vi "Wrap Element To Display.vi"(10 "Camera":refnum<class "Camera.lvclass">, 11 "World Position":T1) -> (3 "Display Position":T1)   [LabVIEW 2018]
uses:
  Camera/Camera.lvclass
  LabSDL2/Source/Libraries/SDL2 Utility/Point (I32).ctl
  Camera/Camera.lvclass/Camera.ctl
  Math/Math.lvlib
  Globals.vi
  Element/Element.lvclass
  LabSDL2/Source/Libraries/SDL2 Utility/SDL2 Utility.lvlib
panel:
  in  "Point":T1
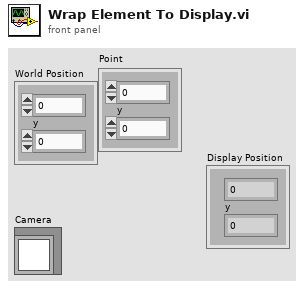
[diagram p1: front panel]
types:
  T1 = typedef "SDL2 Utility.lvlib/Point (I32).ctl" = cluster{"x":i32, "y":i32}
  T2 = typedef "Constants.ctl" = cluster{"Colours":cluster{"OK":u32, "Warning":u32, "Error":u32, "Red":u32, "Green":u32, "Blue":u32, "Yellow":u32}, "System":cluster{"Target Frames Second":dbl, "World Size":T1, "Window Size":T1, "Viewport Size":T1, "Sidebar Scaling":sgl, "Sidebar Width":i32, "SC2 Frame Rate [Seconds/Frame]":sgl}, "Game":cluster{"Maximum Asteroids":i32, "Max Energy":i32, "Max Crew":i32, "Maximum Stars":i32}}
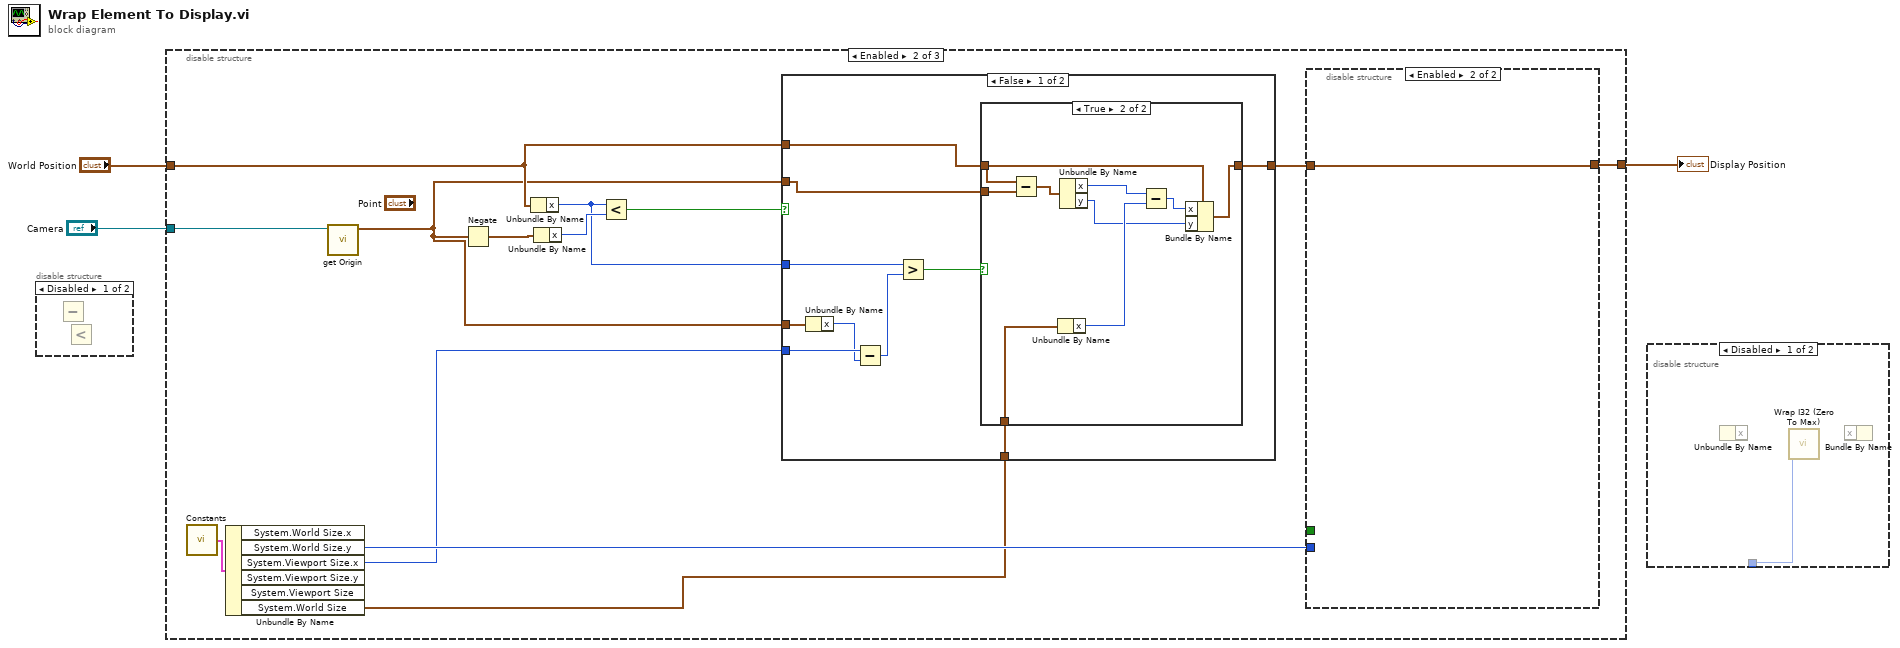
[diagram p0: block diagram]
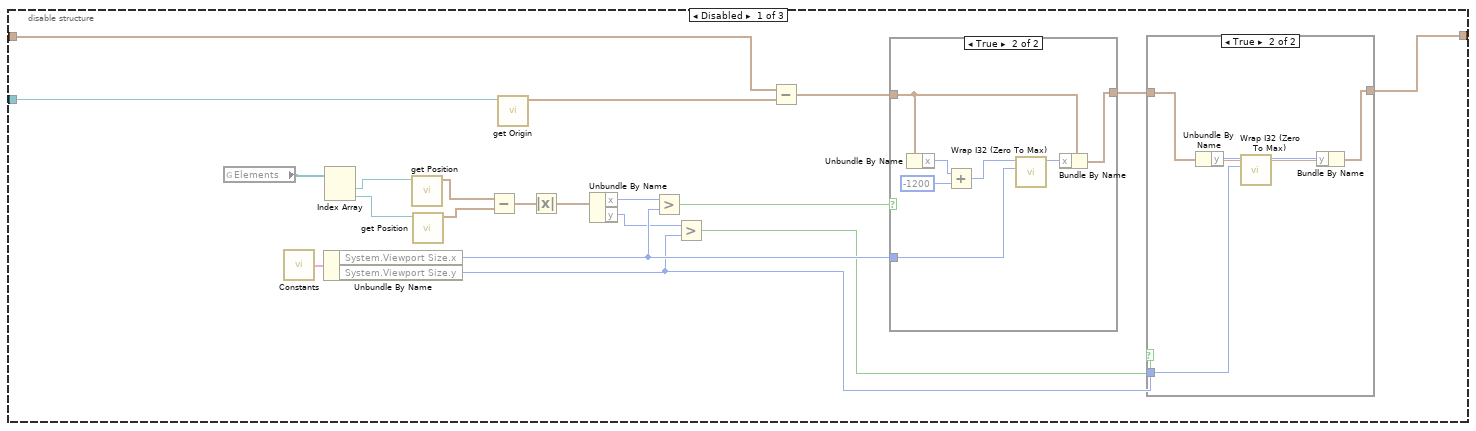
[diagram p4: hidden frame]
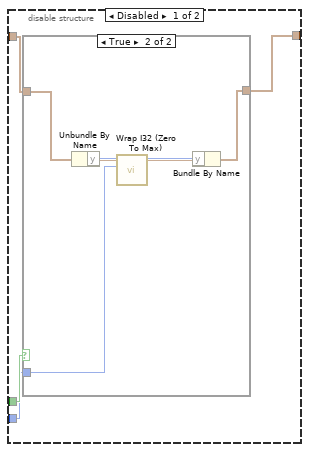
[diagram p7: hidden frame]
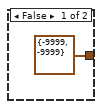
[diagram p9: hidden frame]
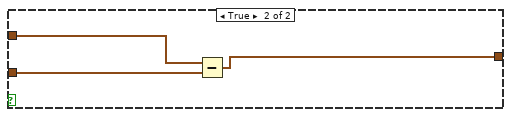
[diagram p10: hidden frame]
diagram:
  n1 = disable-structure shown="Disabled" {
    frame Disabled {
      n2 = Subtract() -> ()  [unwired: 2 in, 1 out]
      n3 = Less?() -> ()  [unwired: 2 in, 1 out]
    }
    frame Enabled {
    }
  }
  n4 = disable-structure shown="Enabled" {
    disable-tunnel: "Camera" -> [w8 w48 _]
    disable-tunnel: [w7 w47 _] -> w2
    disable-tunnel: "World Position" -> [w6 w46 _]
    frame Disabled {
      n5 = global read "Globals.vi" "Elements"() -> (w23:refnum<class "Element.lvclass">[])
      n6 = call "Constants.vi"() -> ("Constants"=w17:T2)
      n7 = Unbundle By Name(w17) -> ("System.Viewport Size.x"=w15:i32, "System.Viewport Size.y"=w9:i32)
      n8 = Index Array(array=w23) -> (element #1=w22:refnum<class "Element.lvclass">, element #2=w21:refnum<class "Element.lvclass">)  [unwired: 2 in]
      n9 = call "get Position.vi"("Movable in"=w22) -> ("Position"=w5:T1)  [unwired: 10 in]
      n10 = call "get Position.vi"("Movable in"=w21) -> ("Position"=w20:T1)  [unwired: 10 in]
      n11 = Subtract(x=w5, y=w20) -> (x-y=w19:T1)
      n12 = call "get Origin.vi"("Camera in"=w8) -> ("Point"=w14:T1)  [unwired: 10 in]
      n13 = Absolute Value(x=w19) -> (abs(x)=w4:T1)
      n14 = Unbundle By Name(w4) -> ("x"=w18:i32, "y"=w11:i32)
      n15 = Greater?(x=w18, y=w15) -> (0:w16:bool)
      n16 = Greater?(x=w11, y=w9) -> (0:w10:bool)
      n17 = Subtract(x=w6, y=w14) -> (x-y=w13:T1)
      n18 = case shown="True" w16 {
        tunnel: [w30 w35] -> w12
        tunnel: w15 -> [_ w36]
        tunnel: w13 -> [w30 w34]
        frame False {
        }
        frame True {
          n19 = Unbundle By Name(w34) -> ("x"=w32:i32)
          n20 = Add(x=w32, y=-1200) -> (x+y=w31:i32)
          n21 = call "Wrap I32 (Zero To Max).vi"("Max"=w36, "Value"=w31) -> ("Wrapped"=w37:i32)  [unwired: 9 in]
          n22 = Bundle By Name(cluster=w34, "x"=w37) -> (w35:T1)
        }
      }
      n23 = case shown="True" w10 {
        tunnel: [w24 w26] -> w7
        tunnel: w12 -> [w24 w27]
        tunnel: w9 -> [_ w25]
        frame False {
        }
        frame True {
          n24 = Unbundle By Name(w27) -> ("y"=w28:i32)
          n25 = call "Wrap I32 (Zero To Max).vi"("Max"=w25, "Value"=w28) -> ("Wrapped"=w29:i32)  [unwired: 9 in]
          n26 = Bundle By Name(cluster=w27, "y"=w29) -> (w26:T1)
        }
      }
    }
    frame Enabled {
      n27 = call "Constants.vi"() -> ("Constants"=w50:T2)
      n28 = Unbundle By Name(w50) -> ("System.World Size.y"=w49:i32, "System.Viewport Size.x"=w40:i32, "System.World Size"=w39:T1)  [unwired: 3 out]
      n29 = call "get Origin.vi"("Camera in"=w48) -> ("Point"=w38:T1)  [unwired: 10 in]
      n30 = Negate(x=w38) -> (-x=w45:T1)
      n31 = Unbundle By Name(w46) -> ("x"=w41:i32)
      n32 = Unbundle By Name(w45) -> ("x"=w44:i32)
      n33 = Less?(x=w41, y=w44) -> (x < y?=w42:bool)
      n34 = case shown="False" w42 {
        tunnel: [w70 w82] -> w43
        tunnel: w46 -> [w71 w83]
        tunnel: w38 -> [w63 w84]
        tunnel: w41 -> [w69 _]
        tunnel: w40 -> [w68 _]
        tunnel: w38 -> [w67 _]
        tunnel: w39 -> [w62 _]
        frame False {
          n35 = Unbundle By Name(w67) -> ("x"=w66:i32)
          n36 = Subtract(x=w68, y=w66) -> (x-y=w65:i32)
          n37 = Greater?(x=w69, y=w65) -> (0:w64:bool)
          n38 = case shown="True" w64 {
            tunnel: w71 -> [_ w80]
            tunnel: [T1 {"x"=-9999, "y"=-9999} ("World Position") w74] -> w70
            tunnel: w63 -> [_ w81]
            tunnel: w62 -> [_ w77]
            frame False {
            }
            frame True {
              n39 = Subtract(x=w80, y=w81) -> (x-y=w79:T1)
              n40 = Unbundle By Name(w77) -> ("x"=w76:i32)
              n41 = Unbundle By Name(w79) -> ("x"=w78:i32, "y"=w73:i32)
              n42 = Subtract(x=w78, y=w76) -> (x-y=w75:i32)
              n43 = Bundle By Name(cluster=w80, "x"=w75, "y"=w73) -> (w74:T1)
            }
          }
        }
        frame True {
          n44 = Subtract(x=w83, y=w84) -> (x-y=w82:T1)
        }
      }
      n45 = disable-structure shown="Enabled" {
        disable-tunnel: w43 -> [w54 w61]
        disable-tunnel: _ -> [w53 _]
        disable-tunnel: w49 -> [w52 _]
        disable-tunnel: [w51 w61] -> w47
        frame Disabled {
          n46 = case shown="True" w53 {
            tunnel: [w55 w57] -> w51
            tunnel: w54 -> [w55 w58]
            tunnel: w52 -> [_ w56]
            frame False {
            }
            frame True {
              n47 = Unbundle By Name(w58) -> ("y"=w59:i32)
              n48 = call "Wrap I32 (Zero To Max).vi"("Max"=w56, "Value"=w59) -> ("Wrapped"=w60:i32)  [unwired: 9 in]
              n49 = Bundle By Name(cluster=w58, "y"=w60) -> (w57:T1)
            }
          }
        }
        frame Enabled {
        }
      }
    }
    frame Disabled {
    }
  }
  "Display Position" <- w2
  n50 = disable-structure shown="Disabled" {
    disable-tunnel: _ -> [w85 _]
    frame Disabled {
      n51 = Unbundle By Name() -> ()  [unwired: 1 in, 1 out]
      n52 = call "Wrap I32 (Zero To Max).vi"("Max"=w85) -> ()  [unwired: 10 in, 1 out]
      n53 = Bundle By Name() -> ()  [unwired: 2 in, 1 out]
    }
    frame Enabled {
    }
  }
